vi "Enforce array size multiple timestamps.vi"(7 "Timestamps (new)":u64[](array[numeric]), 9 "#bytes per timestamp":i32, 11 "Values (new)":u8[](array[numeric])) -> (3 "Values (new) [padded]":u8[](array[numeric]), 5 "Timestamps (new)":u64[](array[numeric]))   [LabVIEW 2021, in "Ring Buffer Time Series Data.lvlib"]
doc: "This VIM will set a size to the <b>Array In</b> and pass it out as <b>Array Out</b>. This VIM can set a Minimum, or Maximum array size setting <b>Mode</b>. The size is then specified with <b>Size</b>. If elements need to be added or removed they can be processed to at the start of the array or the end. Returned will be the elements that needed to be added or removed to meet the size needs.\n\n-------------\nPackage Information\n\nProduct Name: Hooovahh Array VIMs\nPackage File Name: Hooovahh_Array_VIMs-2.1.1.12\nPackage Version: 2.1.1.12\nMinimum LabVIEW Version: 18.0"
uses:
  Ring Buffer Time Series Data.lvlib
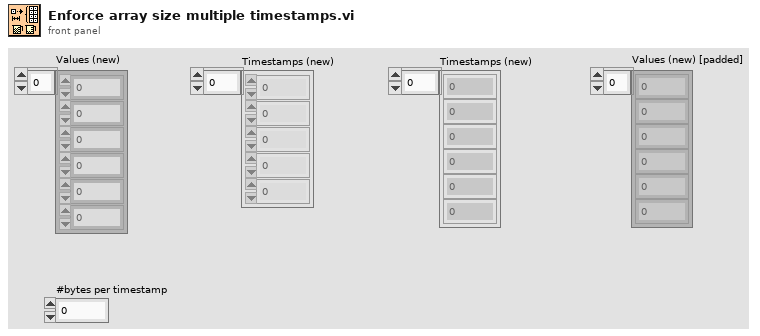
[diagram p1: front panel]
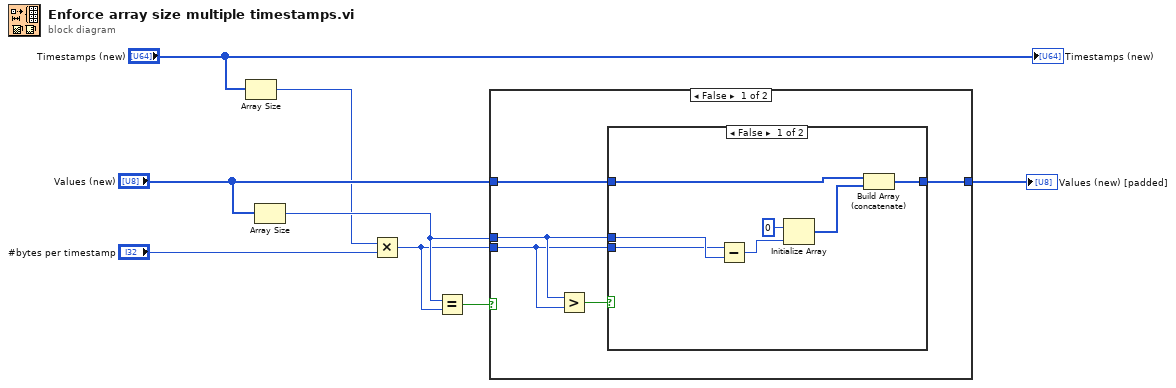
[diagram p0: block diagram]
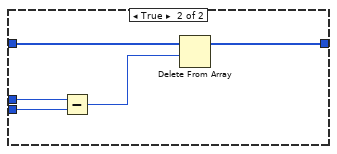
[diagram p2: hidden frame]
diagram:
  n1 = Array Size(array="Timestamps (new)") -> (size(s)=w3:i32)
  n2 = Array Size(array="Values (new)") -> (size(s)=w6:i32)
  n3 = Multiply(x=w3, y="#bytes per timestamp") -> (x*y=w1:i32)
  n4 = Equal?(x=w6, y=w1) -> (x = y?=w5:bool)
  n5 = case shown="False" w5 {
    tunnel: "Values (new)" -> [w13 w26]
    tunnel: [w12 w26] -> w7
    tunnel: w6 -> [w10 _]
    tunnel: w1 -> [w9 _]
    frame False {
      n6 = Greater?(x=w10, y=w9) -> (0:w11:bool)
      n7 = case shown="False" w11 {
        tunnel: w10 -> [w19 w25]
        tunnel: w9 -> [w18 w24]
        tunnel: w13 -> [w15 w23]
        tunnel: [w17 w22] -> w12
        frame False {
          n8 = Subtract(x=w18, y=w19) -> (x-y=w20:i32)
          n9 = Initialize Array(u8 0 ("element"), w20) -> (w14:u8[])
          n10 = Build Array (concatenate)(w15, w14) -> (w17:u8[])
        }
        frame True {
          n11 = Subtract(x=w25, y=w24) -> (x-y=w21:i32)
          n12 = Delete From Array(array=w23, length=w21) -> (array with subset deleted=w22:u8[])  [unwired: 1 in, 1 out]
        }
      }
    }
    frame True {
    }
  }
  "Values (new) [padded]" <- w7
  "Timestamps (new)" <- "Timestamps (new)"
